vi "load_testprofile_registers.vi"(7 "error in (no error)":errorcluster, 9 "path":path=path "C:/Users/christian.acosta/Documents/Projects dev/Stations/Dependencies/TestProfile_OP60_GreyWall_Rev2p3.csv", 10 "index (row)":i32) -> (0 "error out":errorcluster, 2 "subarray":dbl[](array[numeric]), 3 "Numeric":i32)   [LabVIEW 2018]
uses:
  SupportVIs/Read Delimited Spreadsheet (string).vi
panel:
  out "array count":i32
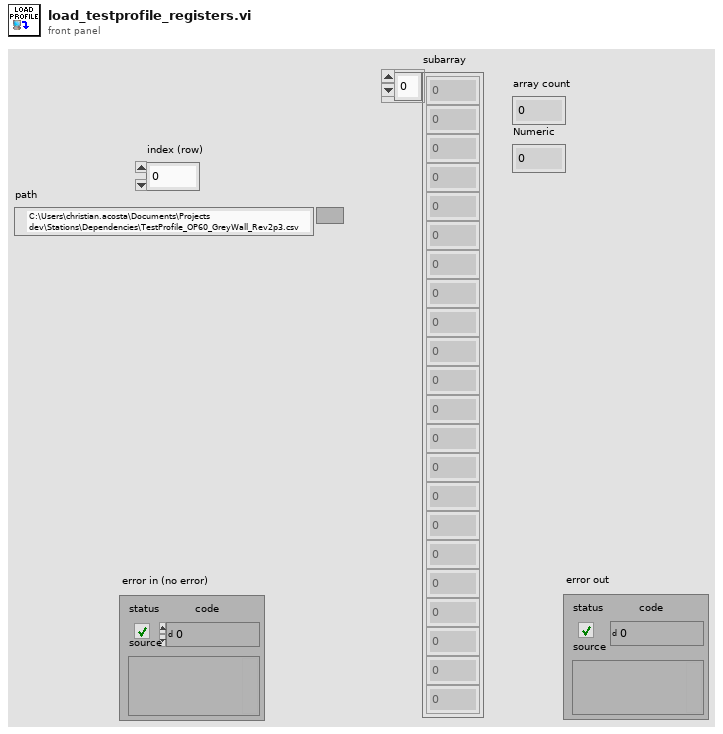
[diagram p1: front panel]
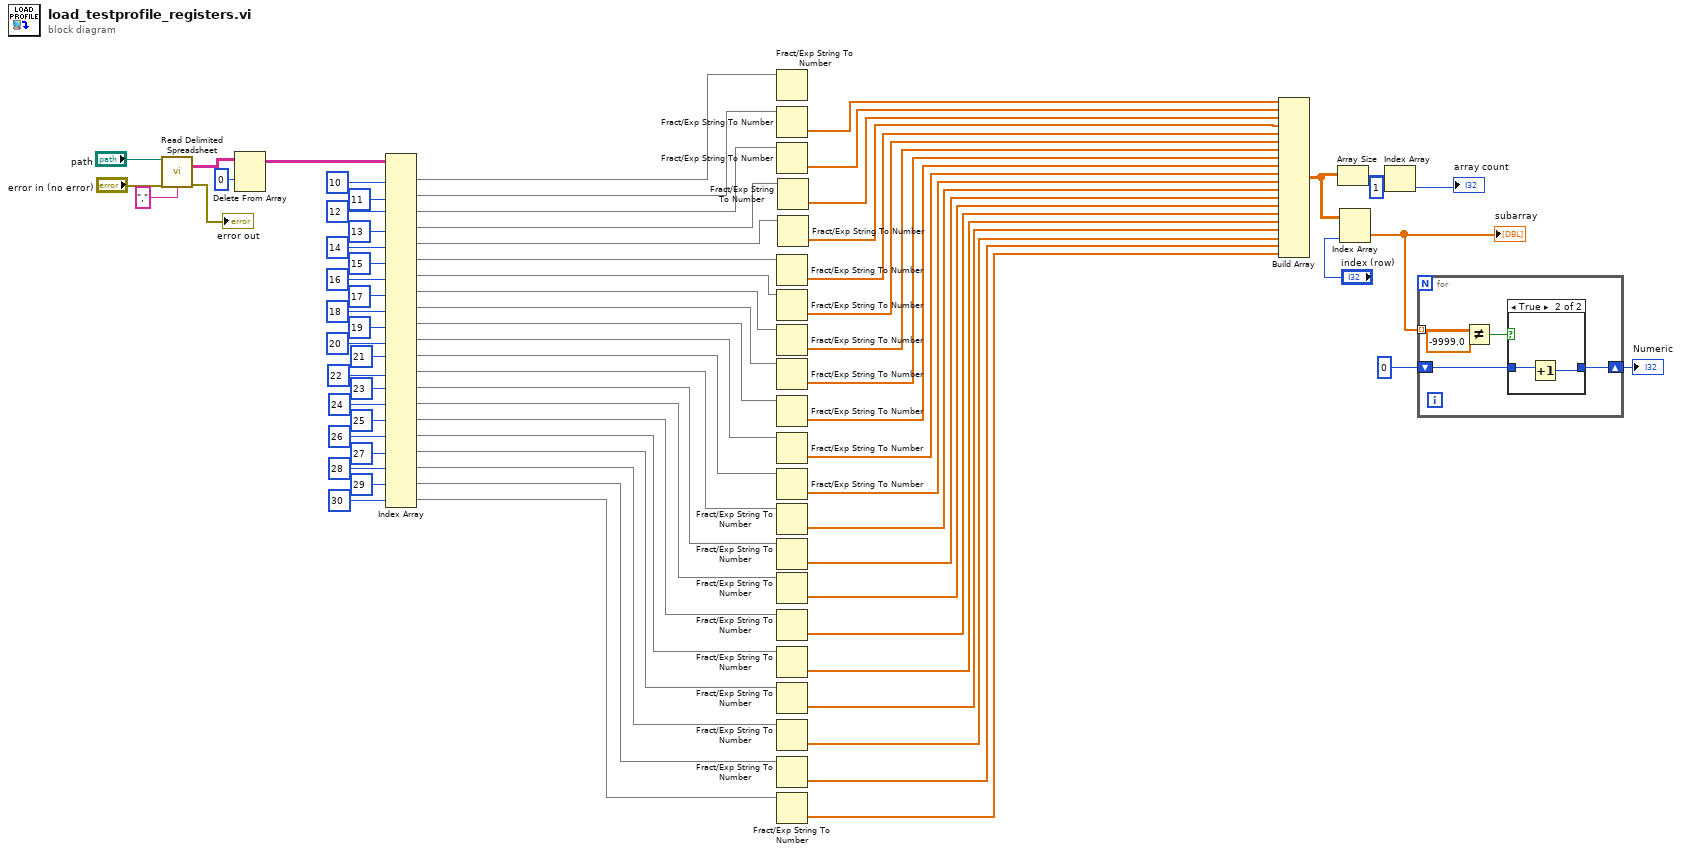
[diagram p0: block diagram]
diagram:
  n1 = call-poly "Read Delimited Spreadsheet.vi"("file path (dialog if empty)"="path", "error in (no error)"="error in (no error)", "delimiter (\\t)"="," ("delimiter (\\t)")) -> ("all rows"=w75:string[][], "error out"=→"error out":errorcluster)  [unwired: 7 in, 4 out]
  n2 = Delete From Array(array=w75, index (row)=0) -> (array with subset deleted=w73:string[][])  [unwired: 2 in, 1 out]
  n3 = Index Array(array=w73, index (col) #1=10 ("disabled index (col)"), index (col) #2=11 ("disabled index (col)"), index (col) #3=12 ("disabled index (col)"), index (col) #4=13 ("disabled index (col)"), index (col) #5=14 ("disabled index (col)"), index (col) #6=15 ("disabled index (col)"), index (col) #7=16 ("disabled index (col)"), index (col) #8=17 ("disabled index (col)"), index (col) #9=18 ("disabled index (col)"), index (col) #10=19 ("disabled index (col)"), index (col) #11=20 ("index (col)"), index (col) #12=21 ("disabled index (col)"), index (col) #13=22 ("disabled index (col)"), index (col) #14=23 ("disabled index (col)"), index (col) #15=24 ("disabled index (col)"), index (col) #16=25 ("disabled index (col)"), index (col) #17=26 ("disabled index (col)"), index (col) #18=27 ("disabled index (col)"), index (col) #19=28 ("disabled index (col)"), index (col) #20=29 ("disabled index (col)"), index (col) #21=30 ("index (col)")) -> (element #1=w71:string[], element #2=w70:string[], element #3=w69:string[], element #4=w4:string[], element #5=w3:string[], element #6=w68:string[], element #7=w67:string[], element #8=w66:string[], element #9=w65:string[], element #10=w64:string[], element #11=w42:string[], element #12=w27:string[], element #13=w26:string[], element #14=w25:string[], element #15=w24:string[], element #16=w23:string[], element #17=w22:string[], element #18=w21:string[], element #19=w20:string[], element #20=w19:string[], element #21=w18:string[])  [unwired: 21 in]
  n4 = Fract/Exp String To Number(string=w71) -> ()  [unwired: 3 in, 2 out]
  n5 = Fract/Exp String To Number(string=w70) -> (number=w63:dbl[])  [unwired: 3 in, 1 out]
  n6 = Fract/Exp String To Number(string=w69) -> (number=w62:dbl[])  [unwired: 3 in, 1 out]
  n7 = Fract/Exp String To Number(string=w68) -> (number=w61:dbl[])  [unwired: 3 in, 1 out]
  n8 = Fract/Exp String To Number(string=w67) -> (number=w60:dbl[])  [unwired: 3 in, 1 out]
  n9 = Fract/Exp String To Number(string=w66) -> (number=w59:dbl[])  [unwired: 3 in, 1 out]
  n10 = Fract/Exp String To Number(string=w65) -> (number=w58:dbl[])  [unwired: 3 in, 1 out]
  n11 = Fract/Exp String To Number(string=w64) -> (number=w57:dbl[])  [unwired: 3 in, 1 out]
  n12 = Fract/Exp String To Number(string=w42) -> (number=w41:dbl[])  [unwired: 3 in, 1 out]
  n13 = Fract/Exp String To Number(string=w27) -> (number=w17:dbl[])  [unwired: 3 in, 1 out]
  n14 = Fract/Exp String To Number(string=w26) -> (number=w16:dbl[])  [unwired: 3 in, 1 out]
  n15 = Fract/Exp String To Number(string=w25) -> (number=w15:dbl[])  [unwired: 3 in, 1 out]
  n16 = Fract/Exp String To Number(string=w24) -> (number=w14:dbl[])  [unwired: 3 in, 1 out]
  n17 = Fract/Exp String To Number(string=w23) -> (number=w13:dbl[])  [unwired: 3 in, 1 out]
  n18 = Fract/Exp String To Number(string=w22) -> (number=w12:dbl[])  [unwired: 3 in, 1 out]
  n19 = Fract/Exp String To Number(string=w21) -> (number=w11:dbl[])  [unwired: 3 in, 1 out]
  n20 = Fract/Exp String To Number(string=w20) -> (number=w10:dbl[])  [unwired: 3 in, 1 out]
  n21 = Fract/Exp String To Number(string=w19) -> (number=w9:dbl[])  [unwired: 3 in, 1 out]
  n22 = Fract/Exp String To Number(string=w18) -> (number=w8:dbl[])  [unwired: 3 in, 1 out]
  n23 = Fract/Exp String To Number(string=w4) -> (number=w2:dbl[])  [unwired: 3 in, 1 out]
  n24 = Fract/Exp String To Number(string=w3) -> (number=w1:dbl[])  [unwired: 3 in, 1 out]
  n25 = Build Array(w63, w62, w2, w1, w61, w60, w59, w58, w57, w41, w17, w16, w15, w14, w13, w12, w11, w10, w9, w8) -> (w40:dbl[][])
  n26 = Array Size(array=w40) -> (size(s)=w44:i32[])
  n27 = Index Array(array=w40, index (col)="index (row)") -> (element=w7:dbl[])  [unwired: 1 in]
  "subarray" <- w7
  n28 = Index Array(array=w44, index=1) -> (element=→"array count":i32)
  n29 = for {
    tunnel: w7 -> [w82] mode=indexing
    shift-right: [w78] -> w5
    shift-left: 0 -> [w79]
    n30 = Not Equal?(x=w82, y=-9999.0) -> (x != y?=w80:bool)
    n31 = case shown="True" w80 {
      tunnel: w79 -> [w83 w85]
      tunnel: [w83 w84] -> w78
      frame False {
      }
      frame True {
        n32 = Increment(x=w85) -> (x+1=w84:i32)
      }
    }
  }
  "Numeric" <- w5
